vi "VIA Per Ranking Results.vi"(8 "error in (no error)":errorcluster, 10 "Ranking Thresholds":T10, 11 "VIAResult":T9 {"Test Config Data"."Test Ranking" items=["Low", "Normal", "High"]}) -> (0 "error out":errorcluster, 2 "Pass?":bool, 3 "Per Ranking Results String":string)   [LabVIEW 2023, in "VIA Results Handling.lvlib"]
doc: "Takes in VIA Results and determines a pass/fail based on Thresholds, per Ranking."
uses:
  VIA Results Handling.lvlib
  <vilib>/addons/analyzer/_analyzerctrls.llb/VIAnCtl Results.ctl
  <vilib>/addons/analyzer/_analyzerctrls.llb/VIAnCtl ResultsData (index).ctl
  <vilib>/addons/analyzer/_analyzerctrls.llb/VIAnCtl ResultStatus.ctl
  <vilib>/addons/analyzer/_vianresshared.llb/VIAnRes Parsed Results Data (by VI).ctl
  <vilib>/addons/analyzer/_vianresshared.llb/VIAnRes Parsed Results Data (by Test).ctl
  <vilib>/addons/analyzer/_analyzerctrls.llb/VIAnCtl Test Config Data.ctl
  <vilib>/addons/analyzer/_analyzerctrls.llb/VIAnCtl TestRanking.ctl
  <vilib>/addons/analyzer/_analyzerctrls.llb/VIAnCtl Config Control Value.ctl
  Ranking Thresholds.ctl
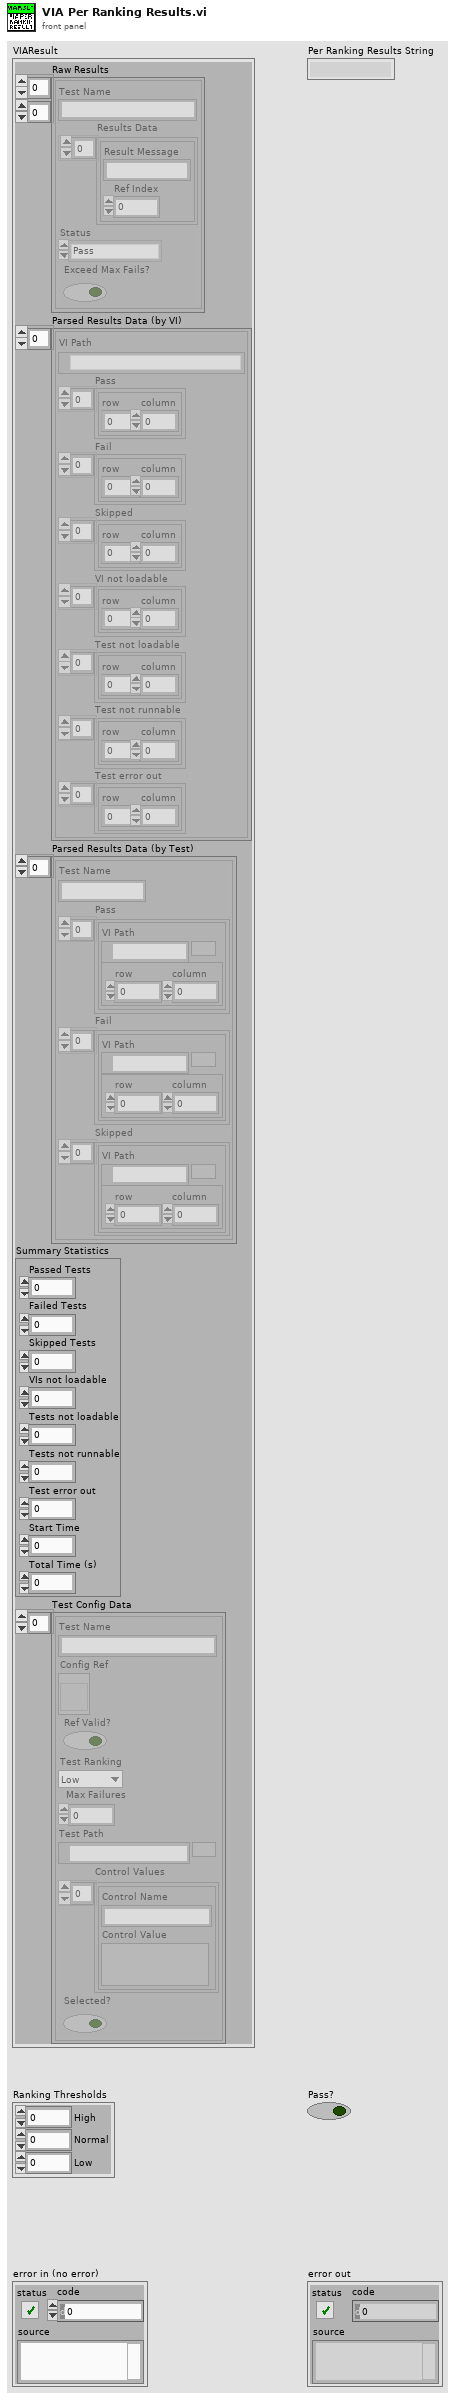
[diagram p1: front panel]
types:
  T1 = typedef "VIAnCtl Results.ctl" = cluster{"Test Name":string, "Results Data":T2[], "Status":T3, "Exceed Max Fails?":bool}
  T2 = typedef "VIAnCtl ResultsData (index).ctl" = cluster{"Result Message":string, "Ref Index":i32}
  T3 = typedef "VIAnCtl ResultStatus.ctl" = enum16{"Pass", "Fail", "Skipped", "VI not loadable", "Test not loadable", "Test not runnable", "Test error out"}
  T4 = typedef "VIAnRes Parsed Results Data (by VI).ctl" = cluster{"VI Path":path, "Pass":cluster{"row":i32, "column":i32}[], "Fail":cluster{"row":i32, "column":i32}[], "Skipped":cluster{"row":i32, "column":i32}[], "VI not loadable":cluster{"row":i32, "column":i32}[], "Test not loadable":cluster{"row":i32, "column":i32}[], "Test not runnable":cluster{"row":i32, "column":i32}[], "Test error out":cluster{"row":i32, "column":i32}[]}
  T5 = typedef "VIAnRes Parsed Results Data (by Test).ctl" = cluster{"Test Name":string, "Pass":cluster{"VI Path":path, "index":cluster{"row":i32, "column":i32}}[], "Fail":cluster{"VI Path":path, "index":cluster{"row":i32, "column":i32}}[], "Skipped":cluster{"VI Path":path, "index":cluster{"row":i32, "column":i32}}[]}
  T6 = typedef "VIAnCtl Test Config Data.ctl" = cluster{"Test Name":string, "Config Ref":refnum<vi>, "Ref Valid?":bool, "Test Ranking":T7, "Max Failures":u32, "Test Path":path, "Control Values":T8[], "Selected?":bool}
  T7 = typedef "VIAnCtl TestRanking.ctl" = u16
  T8 = typedef "VIAnCtl Config Control Value.ctl" = cluster{"Control Name":string, "Control Value":variant}
  T9 = cluster{"Raw Results":T1[][], "Parsed Results Data (by VI)":T4[], "Parsed Results Data (by Test)":T5[], "Summary Statistics":cluster{"Passed Tests":i32, "Failed Tests":i32, "Skipped Tests":i32, "VIs not loadable":i32, "Tests not loadable":i32, "Tests not runnable":i32, "Test error out":i32, "Start Time":u32, "Total Time (s)":dbl}, "Test Config Data":T6[]}
  T10 = typedef "VIA Results Handling.lvlib/Ranking Thresholds.ctl" = cluster{"High":dbl, "Normal":dbl, "Low":dbl}
  T11 = typedef "VIA Results Handling.lvlib/Stats by Ranking.ctl" = cluster{"High":T12, "Normal":T12, "Low":T12}
  T12 = typedef "VIA Results Handling.lvlib/Stats Cluster.ctl" = cluster{"Passed":i32, "Failed":i32, "Skipped":i32, "Total":i32}
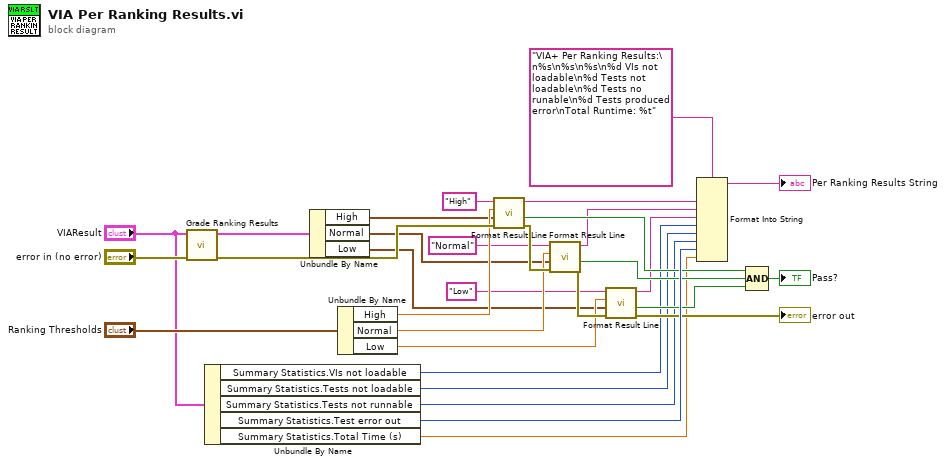
[diagram p0: block diagram]
diagram:
  n1 = call "Grade Ranking Results.vi"("Error in"="error in (no error)", "VIAResult"="VIAResult") -> ("Error out"=w29:errorcluster, "Stats by Ranking"=w23:T11)  [unwired: 8 in]
  n2 = Unbundle By Name("VIAResult") -> ("Summary Statistics.VIs not loadable"=w19:i32, "Summary Statistics.Tests not loadable"=w20:i32, "Summary Statistics.Tests not runnable"=w21:i32, "Summary Statistics.Test error out"=w31:i32, "Summary Statistics.Total Time (s)"=w22:dbl)
  n3 = Unbundle By Name(w23) -> ("High"=w4:T12, "Normal"=w7:T12, "Low"=w8:T12)
  n4 = Unbundle By Name("Ranking Thresholds") -> ("High"=w10:dbl, "Normal"=w11:dbl, "Low"=w12:dbl)
  n5 = call "Format Result Line.vi"("Error in"=w29, "Stats"=w4, "Threshold %"=w10, "Rank"="High") -> ("Error out"=w16:errorcluster, "Pass?"=w24:bool, "Results Description"=w13:string)  [unwired: 5 in]
  n6 = call "Format Result Line.vi"("Error in"=w16, "Stats"=w7, "Threshold %"=w11, "Rank"="Normal") -> ("Error out"=w17:errorcluster, "Pass?"=w25:bool, "Results Description"=w14:string)  [unwired: 5 in]
  n7 = call "Format Result Line.vi"("Error in"=w17, "Stats"=w8, "Threshold %"=w12, "Rank"="Low") -> ("Error out"=→"error out":errorcluster, "Pass?"=w26:bool, "Results Description"=w15:string)  [unwired: 5 in]
  n8 = Format Into String(format string="VIA+ Per Ranking Results:\n%s\n%s\n%s\n%d VIs not loadable\n%d Tests not loadable\n%d Tests no runable\n%d Tests produced error\nTotal Runtime: %t", w13, w14, w15, w19, w20, w21, w31, w22) -> (resulting string=→"Per Ranking Results String":string)  [unwired: 2 in, 1 out]
  n9 = Compound Arithmetic op=AND(w24, w25, w26) -> (→"Pass?":bool)
